vi "averager.vi"(11 "input":dbl[](array[numeric])) -> (3 "output":dbl[](array[numeric]))   [LabVIEW 2014]
uses:
  <vilib>/Analysis/baseanly.llb/Mean (DBL).vi
  <vilib>/Analysis/NI_AALBase.lvlib
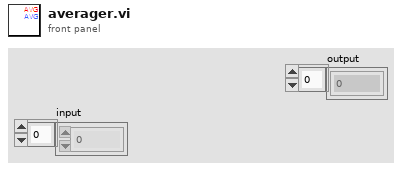
[diagram p1: front panel]
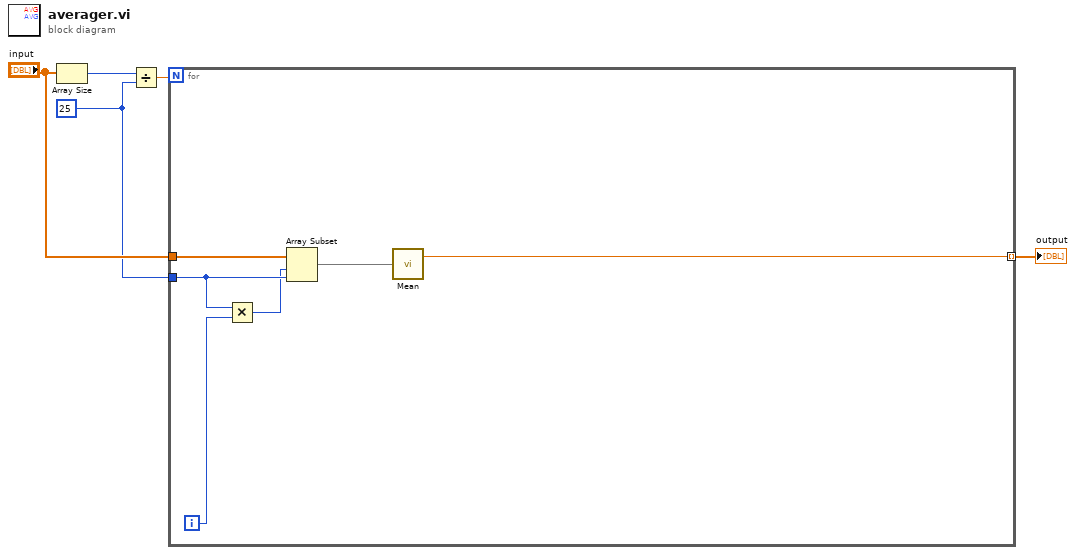
[diagram p0: block diagram]
diagram:
  w2 = 25
  n1 = Array Size(array="input") -> (size(s)=w4:i32)
  n2 = Divide(x=w4, y=w2) -> (x/y=w5:dbl)
  n3 = for {
    N: w5 -> [_]
    tunnel: "input" -> [w11]
    tunnel: w2 -> [w10]
    tunnel: [w6] -> w1 mode=indexing
    i -> [w9]
    n4 = Multiply(x=w10, y=w9) -> (x*y=w8:i32)
    n5 = Array Subset(array=w11, index=w8, length=w10) -> (w7:dbl[])
    n6 = call-poly <vilib>:"Mean.vi"("X"=w7) -> ("mean"=w6:dbl)  [unwired: 1 out]
  }
  "output" <- w1
